vi "Logger.Variant.CompareFiles.vi"() -> ()   [LabVIEW 2016]
uses:
  Logger.Variant.Sets.ctl
  Station/Station.Changeover.State.vi
  Station/Station.Plate.Properties.ctl
  Sequence/Sequence.Code.SerialFormat.ctl
  Drivers/V7310/LowLevel/V7310.Job.Sets.ctl
panel:
  out "Array":T1[](array[typedef])
  in  "Missing items":i32(listbox)
  in  "Diferences":i32(listbox)
  out "size(s) old":i32
  out "size(s) new":i32
  out "size(s) 2":i32
  out "size(s)":i32
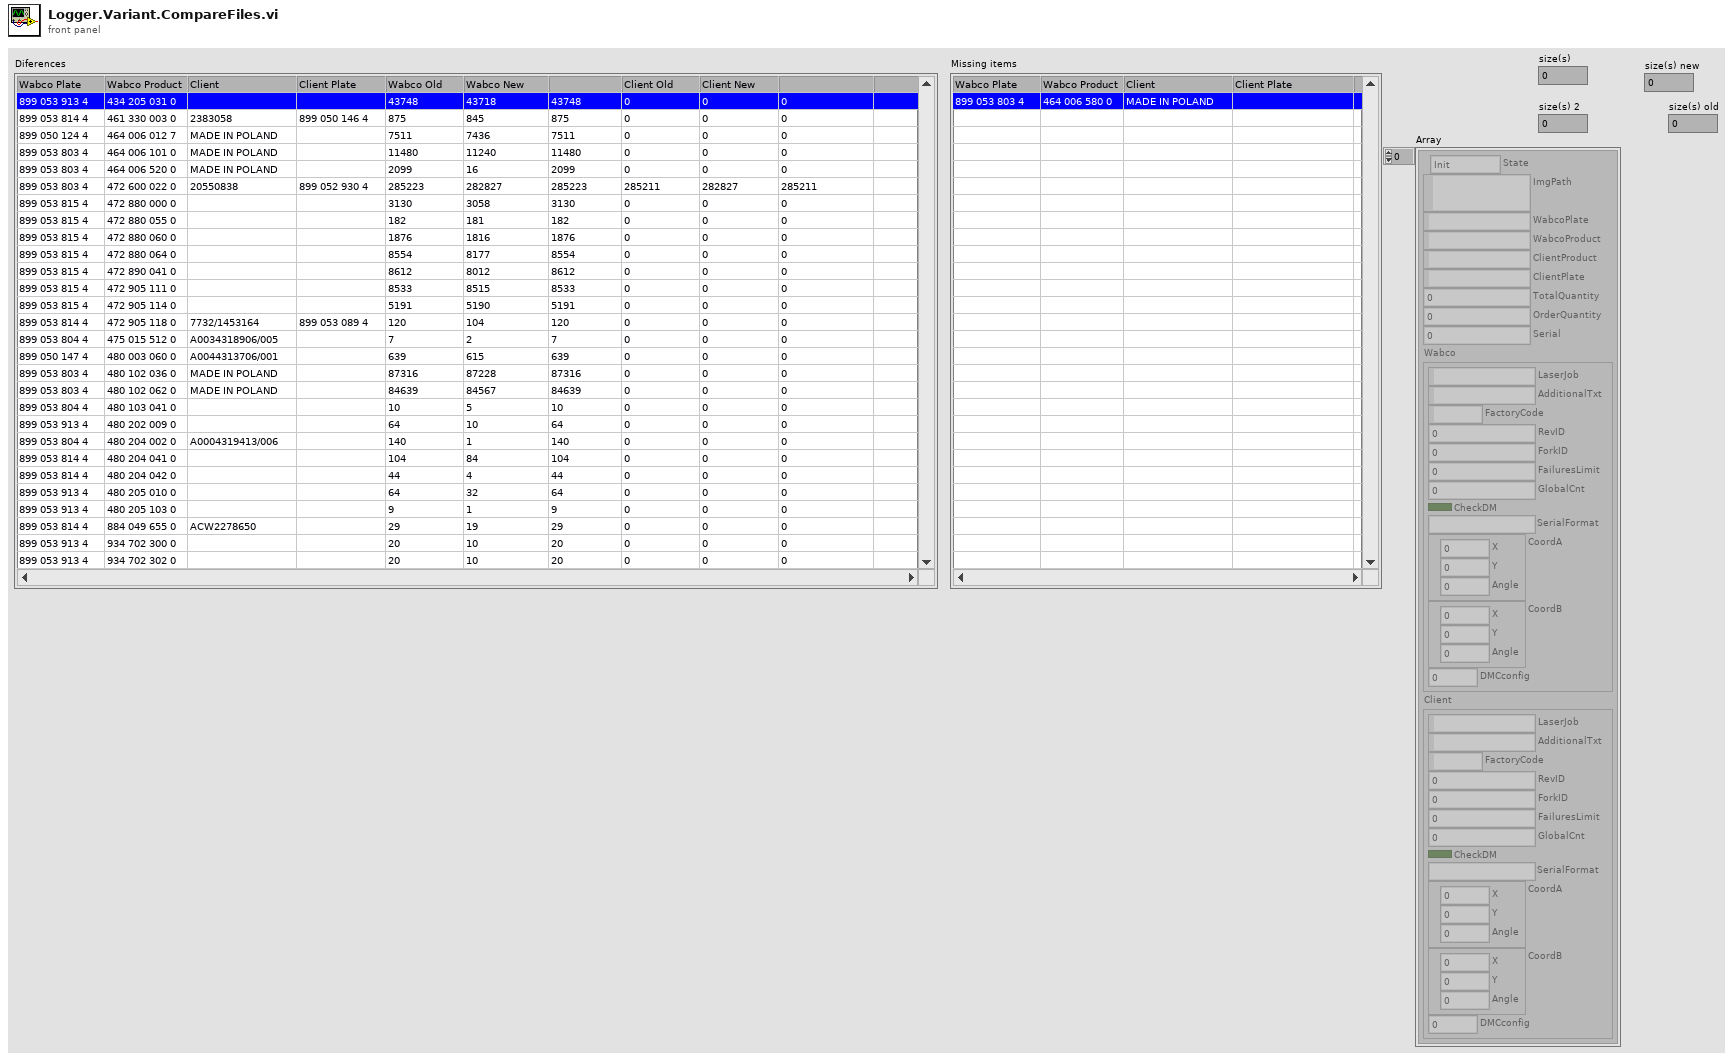
[diagram p1: front panel]
types:
  T1 = typedef "Logger.Variant.Sets.ctl" = cluster{"State":T2, "ImgPath":path, "WabcoPlate":string, "WabcoProduct":string, "ClientProduct":string, "ClientPlate":string, "TotalQuantity":u16, "OrderQuantity":u16, "Serial":i32, "Wabco":T3, "Client":T3}
  T2 = typedef "Station.Changeover.State.vi" = enum16{"Init", "Scaning", "NOK", "Wait for ack", "Ready"}
  T3 = typedef "Station.Plate.Properties.ctl" = cluster{"LaserJob":string, "AdditionalTxt":string, "FactoryCode":string, "RevID":u8, "ForkID":u8, "FailuresLimit":u16, "GlobalCnt":i32, "CheckDM":bool, "SerialFormat":T4, "CoordA":T5, "CoordB":T5, "DMCconfig":i32}
  T4 = typedef "Sequence.Code.SerialFormat.ctl" = enum8{"", "6 dig", "7 dig"}
  T5 = typedef "V7310.Job.Sets.ctl" = cluster{"X":dbl, "Y":dbl, "Angle":dbl}
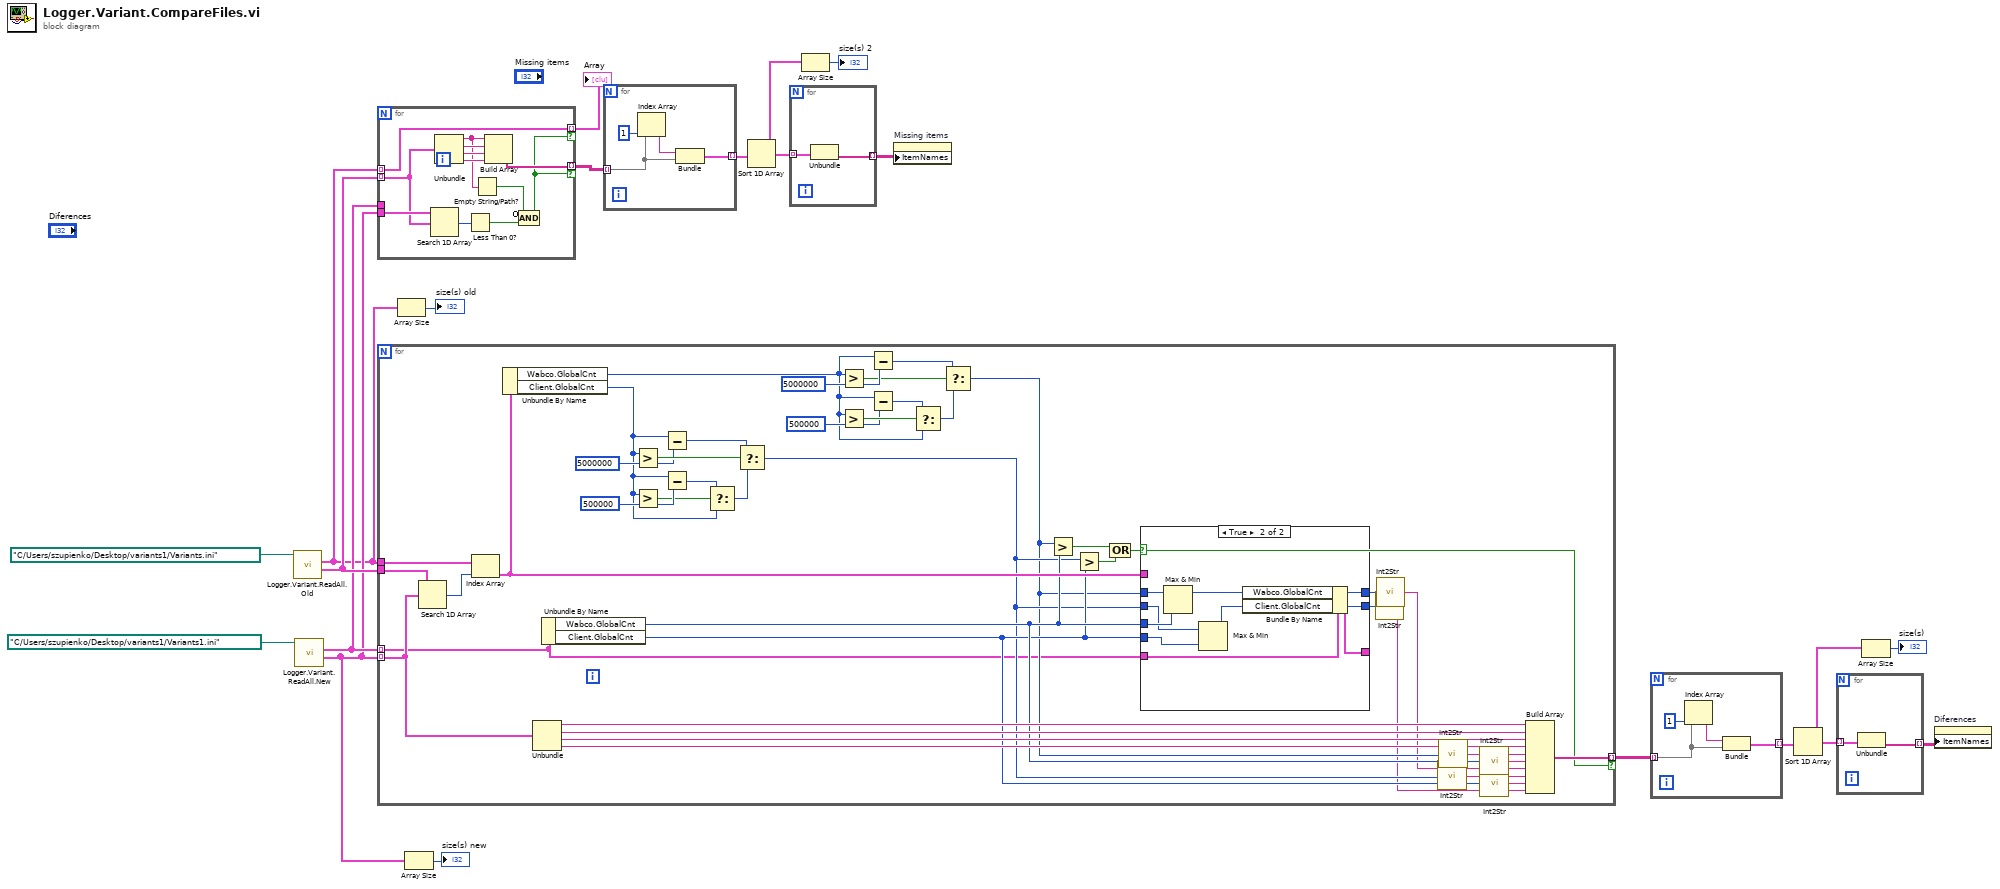
[diagram p0: block diagram]
diagram:
  n1 = call "Logger.Variant.ReadAll.Old.vi"("FilePath"=path "C:/Users/szupienko/Desktop/variants1/Variants.ini") -> ("Orders"=w16:cluster{string, string, string, string}[], "OrdersDetails"=w11:T1[])  [unwired: 8 in, 1 out]
  n2 = call "Logger.Variant.ReadAll.New.vi"("FilePath"=path "C:/Users/szupienko/Desktop/variants1/Variants1.ini") -> ("Orders 2"=w13:cluster{string, string, string, string}[], "OrdersDetails"=w15:T1[])  [unwired: 8 in, 1 out]
  n3 = for {
    tunnel: w16 -> [w29] mode=indexing
    tunnel: w13 -> [w31]
    tunnel: w11 -> [w21] mode=indexing
    tunnel: w15 -> [_]
    tunnel: [w25] -> w5 mode=indexing if=w20
    tunnel: [w21] -> w1 mode=indexing if=w20
    n4 = Search 1D Array(1D array=w31, element=w29) -> (index of element=w30:i32)  [unwired: 1 in]
    n5 = Unbundle(w29) -> (w24:string, w28:string, w27:string, w26:string)
    n6 = Less Than 0?(x=w30) -> (x < 0?=w23:bool)
    n7 = Empty String/Path?(string/path=w24) -> (empty?=w22:bool)
    n8 = Build Array(w24, w28, w27, w26) -> (w25:string[])
    n9 = Compound Arithmetic op=AND(invert w22, w23) -> (w20:bool)
  }
  "Array" <- w1
  n10 = for {
    tunnel: w16 -> [w73]
    tunnel: w13 -> [w68] mode=indexing
    tunnel: w11 -> [w71]
    tunnel: w15 -> [w32] mode=indexing
    tunnel: [w59] -> w10 mode=indexing if=w58
    w45 = 500000 ("y")
    w40 = 5000000 ("y")
    w49 = 500000 ("y")
    w54 = 5000000 ("y")
    n11 = Search 1D Array(1D array=w73, element=w68) -> (index of element=w72:i32)  [unwired: 1 in]
    n12 = Index Array(array=w71, index=w72) -> (element=w57:T1)
    n13 = Unbundle By Name(w57) -> ("Wabco.GlobalCnt"=w48:i32, "Client.GlobalCnt"=w39:i32)
    n14 = Unbundle(w68) -> (w67:string, w66:string, w65:string, w64:string)
    n15 = Unbundle By Name(w32) -> ("Wabco.GlobalCnt"=w56:i32, "Client.GlobalCnt"=w55:i32)
    n16 = Greater?(x=w39, y=w40) -> (0:w41:bool)
    n17 = Greater?(x=w39, y=w45) -> (0:w44:bool)
    n18 = Subtract(x=w39, y=w40) -> (x-y=w42:i32)
    n19 = Subtract(x=w39, y=w45) -> (x-y=w43:i32)
    n20 = Select(t=w43, s=w44, f=w39) -> (s? t:f=w46:i32)
    n21 = Select(t=w42, s=w41, f=w46) -> (s? t:f=w38:i32)
    n22 = Greater?(x=w48, y=w54) -> (0:w53:bool)
    n23 = Greater?(x=w48, y=w49) -> (0:w50:bool)
    n24 = Subtract(x=w48, y=w54) -> (x-y=w52:i32)
    n25 = Subtract(x=w48, y=w49) -> (x-y=w51:i32)
    n26 = Select(t=w51, s=w50, f=w48) -> (s? t:f=w47:i32)
    n27 = Select(t=w52, s=w53, f=w47) -> (s? t:f=w37:i32)
    n28 = Greater?(x=w37, y=w56) -> (0:w70:bool)
    n29 = Greater?(x=w38, y=w55) -> (0:w69:bool)
    n30 = Compound Arithmetic op=OR(w70, w69) -> (w58:bool)
    n31 = case shown="True" w58 {
      tunnel: w32 -> [w76 w84]
      tunnel: w57 -> [_ _]
      tunnel: w37 -> [_ w83]
      tunnel: w56 -> [w75 w82]
      tunnel: w38 -> [_ w81]
      tunnel: w55 -> [w74 w80]
      tunnel: [w76 w79] -> _
      tunnel: [w75 w78] -> w36
      tunnel: [w74 w77] -> w35
      frame False {
      }
      frame True {
        n32 = Max & Min(x=w83, y=w82) -> (max(x,y)=w78:i32)  [unwired: 1 out]
        n33 = Max & Min(x=w81, y=w80) -> (max(x,y)=w77:i32)  [unwired: 1 out]
        n34 = Bundle By Name(cluster=w84, "Wabco.GlobalCnt"=w78, "Client.GlobalCnt"=w77) -> (w79:T1)
      }
    }
    n35 = call "Int2Str.vi"("Numeric"=w35) -> ("string"=w34:string)
    n36 = call "Int2Str.vi"("Numeric"=w36) -> ("string"=w33:string)
    n37 = call "Int2Str.vi"("Numeric"=w38) -> ("string"=w61:string)
    n38 = call "Int2Str.vi"("Numeric"=w37) -> ("string"=w63:string)
    n39 = call "Int2Str.vi"("Numeric"=w56) -> ("string"=w62:string)
    n40 = call "Int2Str.vi"("Numeric"=w55) -> ("string"=w60:string)
    n41 = Build Array(w67, w66, w65, w64, w63, w62, w33, w61, w60, w34) -> (w59:string[])
  }
  n42 = Array Size(array=w11) -> (size(s)=→"size(s) old":i32)
  n43 = Array Size(array=w13) -> (size(s)=→"size(s) new":i32)
  n44 = for {
    tunnel: w5 -> [w86] mode=indexing
    tunnel: [w85] -> w6 mode=indexing
    n45 = Index Array(array=w86, index=1) -> (element=w87:string)
    n46 = Bundle(w87, w86) -> (w85:cluster{string, string[]})  [unwired: 1 in]
  }
  n47 = Sort 1D Array(array=w6) -> (sorted array=w2:cluster{string, string[]}[])
  n48 = for {
    tunnel: w2 -> [w90] mode=indexing
    tunnel: [w89] -> w4 mode=indexing
    n49 = Unbundle(w90) -> (w89:string[])  [unwired: 1 out]
  }
  n50 = Array Size(array=w2) -> (size(s)=→"size(s) 2":i32)
  n51 = property on="Missing items" class="MCListbox (strict)"("ItemNames"=w4) -> ()  [unwired: 2 in, 2 out]
  n52 = for {
    tunnel: w10 -> [w92] mode=indexing
    tunnel: [w91] -> w9 mode=indexing
    n53 = Index Array(array=w92, index=1) -> (element=w93:string)
    n54 = Bundle("string"=w93, w92) -> (w91:cluster{"string":string, string[]})  [unwired: 1 in]
  }
  n55 = Sort 1D Array(array=w9) -> (sorted array=w7:cluster{"string":string, string[]}[])
  n56 = for {
    tunnel: w7 -> [w96] mode=indexing
    tunnel: [w95] -> w8 mode=indexing
    n57 = Unbundle(w96) -> (w95:string[])  [unwired: 1 out]
  }
  n58 = Array Size(array=w7) -> (size(s)=→"size(s)":i32)
  n59 = property on="Diferences" class="MCListbox (strict)"("ItemNames"=w8) -> ()  [unwired: 2 in, 2 out]
